vi "FPGAController_v4.vi"() -> ()   [LabVIEW 2015]
uses:
  <vilib>/Utility/miscctls.llb/LVPointTypeDef.ctl
  <vilib>/FPGAPlugInAG/PXIe-7971R/niLvFpga_Open_PXIe-7971R.vi
  <userlib>/_OpenG.lib/comparison/comparison.llb/DBL Changed__ogtk.vi
  <userlib>/_OpenG.lib/file/file.llb/Strip Path Extension - Path__ogtk.vi
  <userlib>/_OpenG.lib/comparison/comparison.llb/Boolean Changed__ogtk.vi
  <vilib>/Utility/error.llb/Error Cluster From Error Code.vi
  <vilib>/rvi/errors/niLvFpgaAdjustHostInterfaceError.vi
  <vilib>/addons/database/Connection.llb/Conn Execute.vi
  <vilib>/addons/database/Recordset.llb/Rec Fetch Recordset Data (R).vi
  <vilib>/addons/database/Recordset.llb/Rec Destroy - Connection.vi
  <vilib>/FPGAPlugInAG/PXIe-7971R/niLvFpga_Close_PXIe-7971R.vi
  <vilib>/rvi/interface/nirviOpenFPGA/nirviOpenFPGA.xnode
  FPGA Bitfiles/FPGA2_FPGATarget_FPGAcode_ccKM5CyXNW8.lvbitx
  <vilib>/rvi/interface/nirviMethod/nirviMethod.xnode
  <vilib>/FPGA/interface/niFpgaViExecutionMode.ctl
  <vilib>/rvi/interface/nirviReadWriteControl/nirviReadWriteControl.xnode
  <vilib>/addons/database/_DB Variant To Data/Database Variant To Data.xnode
  <vilib>/rvi/interface/nirviCloseFPGA/nirviCloseFPGA.xnode
  <vilib>/addons/database/NI_Database_API.lvlib
  NiFpgaLv.dll
panel:
  out "Time Betwee Shots":dbl
  out "Del Armed":bool
  in  "Lower Threshold":bool
  in  "Raise Threshold":bool
  out "Update Threshold":bool
  in  "Min. Time\nBetween Shots (s)":dbl
  in  "Rate Limiting":bool
  out "Armed":bool
  in  "Add Delay":bool
  in  "Delay Name":string
  in  "Delay Value":dbl=3.0 min=0.0
  in  "Delay Ring":dbl(ring)=3.15039 items=["Ablation Chamber"=6.45, "LEIL Chamber"=4.318, "Third Detector"=3.15039, "Custom"=0.0]
  in  "Rearm Trigger":bool
  in  "One Shot Mode":bool
  out "Last Update:":timestamp
  out "Updating FPGA":bool
  out "Sensitivity":dbl
  out "error out":errorcluster
  out "Low Mass Limit":fxp<+,31,17>
  out "High Mass Limit":fxp<+,31,17>
  out "stopping":bool
  in  "Auto Threshold":bool
  out "Peletron (MV)":dbl=2.0
  out "High Mass (kg)":dbl=inf
  out "Low Mass (kg)":dbl
  out "High Charge Limit":i16
  out "Low Charge Limit":i16
  out "High velocity count":i32=210
  out "Low velocity count":i32=21000
  in  "stop":bool
  in  "Peak-Threshold Factor":dbl=2.0
  out "Low Charge Limit (fC)":dbl
  out "High Charge Limit (fC)":dbl=100.0
  out "High Velocity":dbl=100000.0
  out "Low Velocity":dbl=1000.0
  out "Filter 7 Peak":i32=7483
  out "Filter 6 Peak":i32=9863
  out "Filter 5 Peak":i32=13910
  out "Filter 4 Peak":i32=18191
  out "Filter 3 Peak":i32=46254
  out "Filter 2 Peak":i32=120664
  out "Filter 1 Peak":i32=295996
  in  "Filter7 Threshold":i32=-21165
  in  "Filter6 Threshold":i32=-29358
  in  "Filter5 Threshold":i32=-41730
  in  "Filter4 Threshold":i32=-54306
  in  "Filter3 Threshold":i32=-138762
  in  "Filter2 Threshold":i32=-361992
  in  "Filter1 Threshold":i32=-887988
  in  "Zero Peak Values":bool
  in  "Assign Threshold":bool
  in  "Run Mode":bool
  # "Settings"
  # "Dubugging"
  # "Independent Variable"
  # "Low Vel."
  # "High Vel."
  # "Low Q (fC)"
  # "High Q (fC)"
  # "Plate Control While Loop Counter"
  # "Low Mass (kg)"
  # "High Mass (kg)"
  # "Sens. (V/pC)"
  # "Peletron (MV)"
  # "Current Value of Running Average"
  # "Peak Threshold Factor"
  # "Delay Trigger"
  # "Dist. from 2nd Det. (m)"
  # "Name"
  # "Peak Values"
  # "Peak 1"
  # "Peak 2"
  # "Peak 3"
  # "Peak 4"
  # "Peak 5"
  # "Peak 6"
  # "Peak 7"
  # "Thresholds"
  # "Threshold 1"
  # "Threshold 2"
  # "Threshold 3"
  # "Threshold 4"
  # "Threshold 5"
  # "Threshold 6"
  # "Threshold 7"
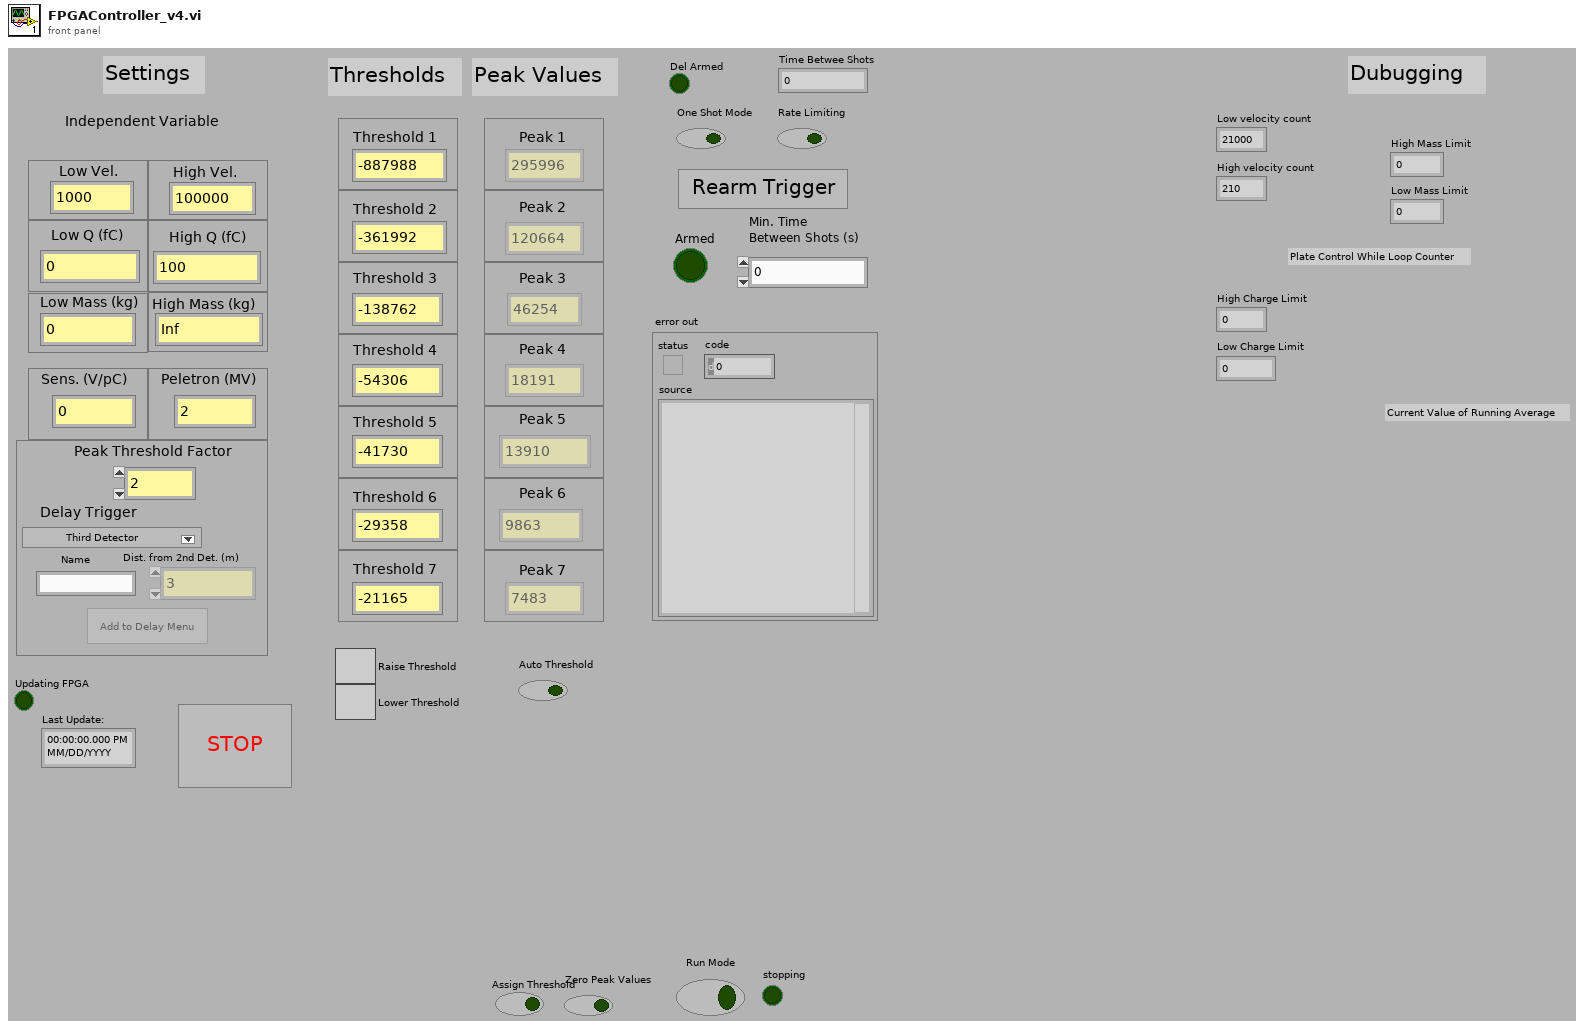
[diagram p1: front panel]
types:
  T1 = typedef "LVPointTypeDef.ctl" = cluster{"Horizontal":i16, "Vertical":i16}
  T2 = enum8{"Enabled", "Disabled", "Disabled and Grayed Out"}
  T3 = typedef "NI_Database_API.lvlib/Conn ObjectReference.ctl" = refnum<k1>
  T4 = cluster{"Filter 1 Peak":i32, "Filter 2 Peak":i32, "Filter 3 Peak":i32, "Filter 4 Peak":i32, "Filter 5 Peak":i32, "Filter 6 Peak":i32, "Filter 7 Peak":i32}
  T5 = typedef "NI_Database_API.lvlib/Rec ObjectReference.ctl" = refnum<k1>
  T6 = typedef "LVStringsAndValuesArrayTypeDef_DBL.ctl" = cluster{"String":string, "Value":dbl}[]
  T7 = cluster{"Numeric":dbl, "Numeric":dbl, "Numeric":dbl, "Numeric":dbl, "Numeric":dbl, "Numeric":dbl, dbl, dbl, "Value":dbl, fxp<+,16,7>, bool}
  T8 = cluster{"Low Velocity Count":i32, "High Velocity Count":i32, "Low Charge Limit (ADC ticks)":i16, "High Charge Limit (ADC ticks)":i16, "Low Mass (ADC*cycle^2)":i64, "High Mass (ADC*cycle^2)":i64, "Mult":fxp<+,16,7>, "Mult Use?":bool}
  T9 = cluster{"Filter 1 Detector 3 Correlation":i32, "Filter 2 Detector 3 Correlation":i32, "Filter 3 Detector 3 Correlation":i32, "Filter 4 Detector 3 Correlation":i32, "Filter 5 Detector 3 Correlation":i32, "Filter 6 Detector 3 Correlation":i32, "Filter 7 Detector 3 Correlation":i32}
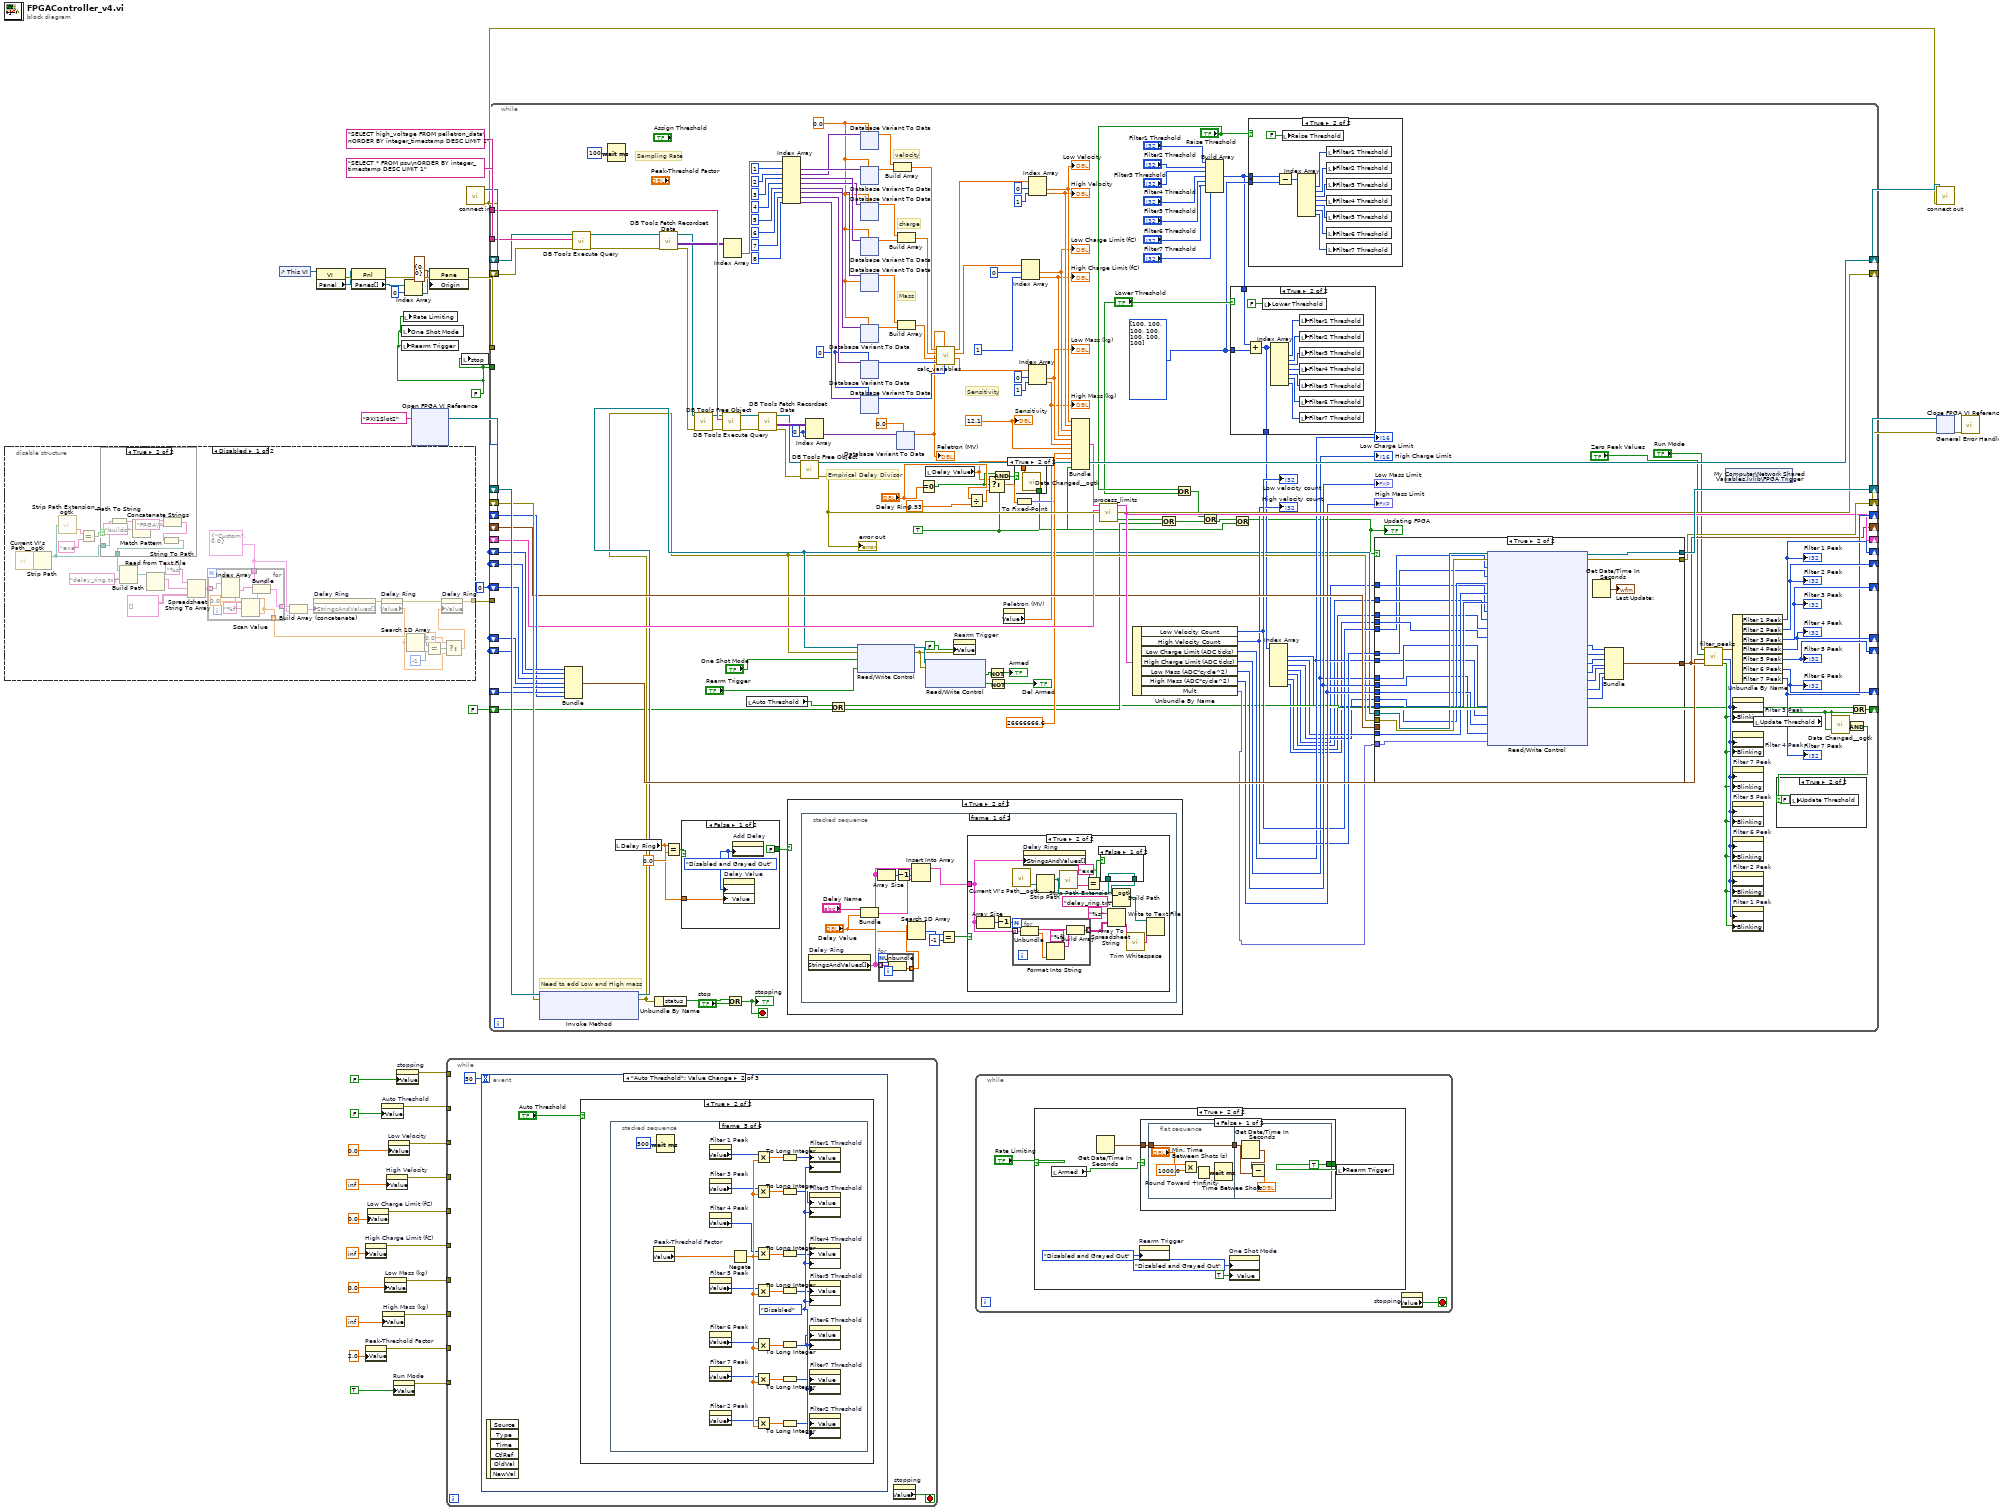
[diagram p0: block diagram]
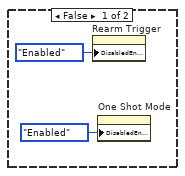
[diagram p4: hidden frame]
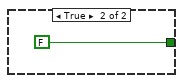
[diagram p5: hidden frame]
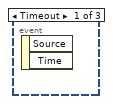
[diagram p6: hidden frame]
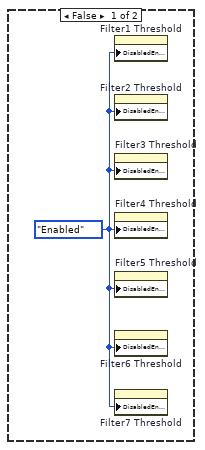
[diagram p7: hidden frame]
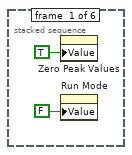
[diagram p8: hidden frame]
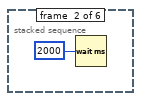
[diagram p9: hidden frame]
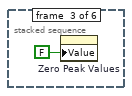
[diagram p10: hidden frame]
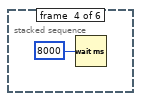
[diagram p11: hidden frame]
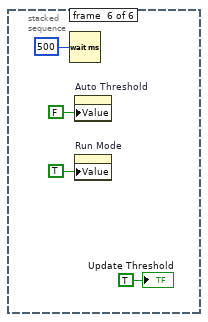
[diagram p12: hidden frame]
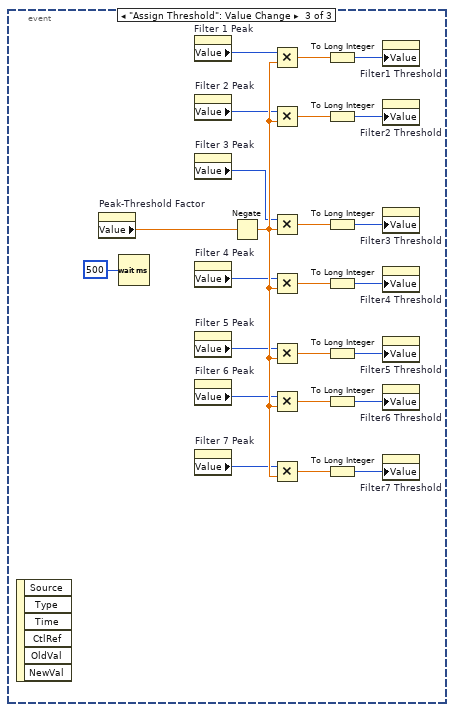
[diagram p13: hidden frame]
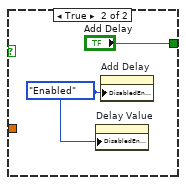
[diagram p18: hidden frame]
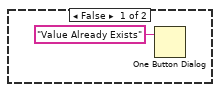
[diagram p20: hidden frame]
diagram:
  w1 = FALSE
  w42 = 0
  n1 = disable-structure shown="Disabled" {
    disable-tunnel: [w50 _] -> w3
    frame Disabled {
      w59 = cluster{"String":string, "Value":dbl} {"String"="Custom", "Value"=0.0}
      n2 = call <userlib>:"Current VI's Path__ogtk.vi"() -> ("Current VI's Path (+ Relative)"=w68:path)  [unwired: 1 in]
      n3 = Strip Path(path=w68) -> (stripped path=w54:path)  [unwired: 1 out]
      n4 = call-poly <userlib>:"Strip Path Extension__ogtk.vi"("path"=w54) -> ("extension"=w58:string)  [unwired: 1 out]
      n5 = Equal?(x=w58, y="exe") -> (x = y?=w55:bool)
      n6 = case shown="True" w55 {
        tunnel: w54 -> [w77 w84]
        tunnel: [w77 w78] -> w53
        frame False {
        }
        frame True {
          n7 = Path To String(path=w84) -> (string=w83:string)
          n8 = Match Pattern(string=w83, regular expression="builds") -> (before substring=w81:string)  [unwired: 1 in, 3 out]
          n9 = Concatenate Strings(w81, "FPGA\\" ("string")) -> (w79:string)
          n10 = String To Path(string=w79) -> (path=w78:path)
        }
      }
      n11 = Build Path(base path=w53, name or relative path="delay_ring.txt") -> (appended path=w56:path)
      n12 = Read from Text File(file (use dialog)=w56) -> (text=w66:string)  [unwired: 3 in, 3 out]
      n13 = Spreadsheet String To Array(format string="%s", spreadsheet string=w66, array type (2D Dbl)=string[][] []) -> (array=w63:string[][])  [unwired: 1 in]
      n14 = for {
        tunnel: w63 -> [w76] mode=indexing
        tunnel: w59 -> [w74]
        tunnel: [w70] -> w60 mode=indexing
        tunnel: [w69] -> w52 mode=indexing
        n15 = Index Array(array=w76) -> (element #1=w75:string, element #2=w73:string)  [unwired: 2 in]
        n16 = Scan Value(string=w73, format string="%f", default (0 dbl)=0.0) -> (value=w69:dbl)  [unwired: 1 out]
        n17 = Bundle(cluster=w74, "String"=w75, "Value"=w69) -> (w70:cluster{"String":string, "Value":dbl})
      }
      n18 = Build Array (concatenate)(w60, w59) -> (w62:cluster{"String":string, "Value":dbl}[])
      n19 = property on="Delay Ring" class="Ring (strict)"("StringsAndValues[]"=w62) -> (error out=w61:errorcluster)  [unwired: 2 in, 1 out]
      n20 = property on="Delay Ring" class="Ring (strict)"(error in=w61) -> (error out=w51:errorcluster, "Value"=w45:dbl)  [unwired: 1 in, 1 out]
      n21 = Search 1D Array(1D array=w52, element=w45) -> (index of element=w49:i32)  [unwired: 1 in]
      n22 = Equal?(x=w49, y=-1) -> (x = y?=w47:bool)
      n23 = Select(t=0.0, s=w47, f=w45) -> (s? t:f=w46:dbl)
      n24 = property on="Delay Ring" class="Ring (strict)"(error in=w51, "Value"=w46) -> (error out=w50:errorcluster)  [unwired: 1 in, 1 out]
    }
    frame Enabled {
    }
  }
  n25 = control-ref of="This VI"() -> (w14:refnum<vi>)
  n26 = property class="VI"(reference=w14) -> (error out=w13:errorcluster, "Panel"=w12:refnum<vi>)  [unwired: 1 in, 1 out]
  n27 = property class="Pnl"(reference=w12, error in=w13) -> (error out=w11:errorcluster, "Panes[]"=w10:refnum<vi>[])  [unwired: 1 out]
  n28 = property on="High Charge Limit (fC)" class="DigNum (strict)"("Value"=inf ("High Charge Limit (fC)")) -> (error out=w29:errorcluster)  [unwired: 2 in, 1 out]
  n29 = property on="Peak-Threshold Factor" class="DigNum (strict)"("Value"=2.0 ("Peak-Threshold Factor")) -> (error out=w23:errorcluster)  [unwired: 2 in, 1 out]
  n30 = property on="Low Charge Limit (fC)" class="DigNum (strict)"("Value"=0.0 ("Low Charge Limit (fC)")) -> (error out=w31:errorcluster)  [unwired: 2 in, 1 out]
  n31 = property on="Auto Threshold" class="Bool (strict)"("Value"=FALSE ("Auto Threshold")) -> (error out=w37:errorcluster)  [unwired: 2 in, 1 out]
  n32 = property on="High Mass (kg)" class="DigNum (strict)"("Value"=inf ("High Mass (kg)")) -> (error out=w25:errorcluster)  [unwired: 2 in, 1 out]
  n33 = property on="Low Mass (kg)" class="DigNum (strict)"("Value"=0.0 ("Low Mass (kg)")) -> (error out=w27:errorcluster)  [unwired: 2 in, 1 out]
  n34 = property on="High Velocity" class="DigNum (strict)"("Value"=inf ("High Velocity")) -> (error out=w33:errorcluster)  [unwired: 2 in, 1 out]
  n35 = property on="Low Velocity" class="DigNum (strict)"("Value"=0.0 ("Low Velocity")) -> (error out=w35:errorcluster)  [unwired: 2 in, 1 out]
  n36 = property on="Run Mode" class="Bool (strict)"("Value"=TRUE ("Run Mode")) -> (error out=w21:errorcluster)  [unwired: 2 in, 1 out]
  n37 = property on="stopping" class="Bool (strict)"("Value"=FALSE ("stopping")) -> (error out=w39:errorcluster)  [unwired: 2 in, 1 out]
  n38 = local write "Rearm Trigger"(w1) -> ()
  n39 = local write "One Shot Mode"(w1) -> ()
  n40 = local write "Rate Limiting"(w1) -> ()
  n41 = Index Array(array=w10, index=0) -> (element=w8:refnum<vi>)
  n42 = xnode "Open FPGA VI Reference"("resource name"=tag "PXI1Slot2") -> ("FPGA VI Reference Out"=w5:refnum<k20>)  [unwired: 1 in, 1 out]
  n43 = property class="Pane"(reference=w8, error in=w11, "Origin"=T1 {"Horizontal"=0, "Vertical"=0}) -> (error out=w6:errorcluster)  [unwired: 1 out]
  n44 = while {
    tunnel: w39 -> [_]
    tunnel: w37 -> [_]
    tunnel: w35 -> [_]
    tunnel: w33 -> [_]
    tunnel: w31 -> [_]
    tunnel: w29 -> [_]
    tunnel: w27 -> [_]
    tunnel: w25 -> [_]
    tunnel: w23 -> [_]
    tunnel: w21 -> [_]
    stop <- w86 stop-if-true
    n45 = event shown="[1] \"Auto Threshold\": Value Change" {
      selector: _ -> [_ _ _]
      dyn-events: _ -> [_ _ _]
      timeout: 50 -> [_ _ _]
      event Timeout {
        n46 = event-data() -> ()  [unwired: 1 in, 2 out]
      }
      event "Auto Threshold": Value Change {
        n47 = event-data() -> ()  [unwired: 1 in, 6 out]
        n48 = case shown="True" "Auto Threshold" {
          frame False {
            w88 = T2."Enabled" ("Disabled")
            n49 = property on="Filter1 Threshold" class="DigNum (strict)"("DisabledEnum"=w88) -> ()  [unwired: 2 in, 2 out]
            n50 = property on="Filter2 Threshold" class="DigNum (strict)"("DisabledEnum"=w88) -> ()  [unwired: 2 in, 2 out]
            n51 = property on="Filter3 Threshold" class="DigNum (strict)"("DisabledEnum"=w88) -> ()  [unwired: 2 in, 2 out]
            n52 = property on="Filter4 Threshold" class="DigNum (strict)"("DisabledEnum"=w88) -> ()  [unwired: 2 in, 2 out]
            n53 = property on="Filter5 Threshold" class="DigNum (strict)"("DisabledEnum"=w88) -> ()  [unwired: 2 in, 2 out]
            n54 = property on="Filter6 Threshold" class="DigNum (strict)"("DisabledEnum"=w88) -> ()  [unwired: 2 in, 2 out]
            n55 = property on="Filter7 Threshold" class="DigNum (strict)"("DisabledEnum"=w88) -> ()  [unwired: 2 in, 2 out]
          }
          frame True {
            n56 = stacked-sequence {
              frame #0 {
                n57 = property on="Zero Peak Values" class="Bool (strict)"("Value"=TRUE ("Zero Peak Values")) -> ()  [unwired: 2 in, 2 out]
                n58 = property on="Run Mode" class="Bool (strict)"("Value"=FALSE ("Run Mode")) -> ()  [unwired: 2 in, 2 out]
              }
              frame #1 {
                n59 = Wait (ms)(milliseconds to wait=u32 2000) -> ()  [unwired: 1 out]
              }
              frame #2 {
                n60 = property on="Zero Peak Values" class="Bool (strict)"("Value"=FALSE ("Zero Peak Values")) -> ()  [unwired: 2 in, 2 out]
              }
              frame #3 {
                n61 = Wait (ms)(milliseconds to wait=u32 8000) -> ()  [unwired: 1 out]
              }
              frame #4 {
                w118 = T2."Disabled" ("Disabled")
                n62 = property on="Peak-Threshold Factor" class="DigNum (strict)"() -> ("Value"=w103:dbl)  [unwired: 2 in, 2 out]
                n63 = Wait (ms)(milliseconds to wait=u32 500) -> ()  [unwired: 1 out]
                n64 = property on="Filter 1 Peak" class="DigNum (strict)"() -> ("Value"=w101:i32)  [unwired: 2 in, 2 out]
                n65 = property on="Filter 3 Peak" class="DigNum (strict)"() -> ("Value"=w99:i32)  [unwired: 2 in, 2 out]
                n66 = property on="Filter 4 Peak" class="DigNum (strict)"() -> ("Value"=w98:i32)  [unwired: 2 in, 2 out]
                n67 = property on="Filter 5 Peak" class="DigNum (strict)"() -> ("Value"=w97:i32)  [unwired: 2 in, 2 out]
                n68 = property on="Filter 6 Peak" class="DigNum (strict)"() -> ("Value"=w96:i32)  [unwired: 2 in, 2 out]
                n69 = property on="Filter 7 Peak" class="DigNum (strict)"() -> ("Value"=w95:i32)  [unwired: 2 in, 2 out]
                n70 = property on="Filter 2 Peak" class="DigNum (strict)"() -> ("Value"=w100:i32)  [unwired: 2 in, 2 out]
                n71 = Negate(x=w103) -> (-x=w102:dbl)
                n72 = Multiply(x=w101, y=w102) -> (x*y=w117:dbl)
                n73 = Multiply(x=w99, y=w102) -> (x*y=w113:dbl)
                n74 = Multiply(x=w98, y=w102) -> (x*y=w111:dbl)
                n75 = Multiply(x=w97, y=w102) -> (x*y=w109:dbl)
                n76 = Multiply(x=w96, y=w102) -> (x*y=w107:dbl)
                n77 = Multiply(x=w95, y=w102) -> (x*y=w105:dbl)
                n78 = Multiply(x=w100, y=w102) -> (x*y=w115:dbl)
                n79 = To Long Integer(number=w117) -> (32bit integer=w116:i32)
                n80 = To Long Integer(number=w113) -> (32bit integer=w112:i32)
                n81 = To Long Integer(number=w111) -> (32bit integer=w110:i32)
                n82 = To Long Integer(number=w109) -> (32bit integer=w108:i32)
                n83 = To Long Integer(number=w107) -> (32bit integer=w106:i32)
                n84 = To Long Integer(number=w105) -> (32bit integer=w104:i32)
                n85 = To Long Integer(number=w115) -> (32bit integer=w114:i32)
                n86 = property on="Filter1 Threshold" class="DigNum (strict)"("Value"=w116, "DisabledEnum"=w118) -> ()  [unwired: 2 in, 2 out]
                n87 = property on="Filter3 Threshold" class="DigNum (strict)"("Value"=w112, "DisabledEnum"=w118) -> ()  [unwired: 2 in, 2 out]
                n88 = property on="Filter4 Threshold" class="DigNum (strict)"("Value"=w110, "DisabledEnum"=w118) -> ()  [unwired: 2 in, 2 out]
                n89 = property on="Filter5 Threshold" class="DigNum (strict)"("Value"=w108, "DisabledEnum"=w118) -> ()  [unwired: 2 in, 2 out]
                n90 = property on="Filter6 Threshold" class="DigNum (strict)"("Value"=w106, "DisabledEnum"=w118) -> ()  [unwired: 2 in, 2 out]
                n91 = property on="Filter7 Threshold" class="DigNum (strict)"("Value"=w104, "DisabledEnum"=w118) -> ()  [unwired: 2 in, 2 out]
                n92 = property on="Filter2 Threshold" class="DigNum (strict)"("Value"=w114, "DisabledEnum"=w118) -> ()  [unwired: 2 in, 2 out]
              }
              frame #5 {
                n93 = Wait (ms)(milliseconds to wait=u32 500) -> ()  [unwired: 1 out]
                n94 = property on="Auto Threshold" class="Bool (strict)"("Value"=FALSE ("Auto Threshold")) -> ()  [unwired: 2 in, 2 out]
                n95 = property on="Run Mode" class="Bool (strict)"("Value"=TRUE ("Run Mode")) -> ()  [unwired: 2 in, 2 out]
                "Update Threshold" <- TRUE ("Update Threshold")
              }
            }
          }
        }
      }
      event "Assign Threshold": Value Change {
        n96 = event-data() -> ()  [unwired: 1 in, 6 out]
        n97 = property on="Peak-Threshold Factor" class="DigNum (strict)"() -> ("Value"=w137:dbl)  [unwired: 2 in, 2 out]
        n98 = Wait (ms)(milliseconds to wait=u32 500) -> ()  [unwired: 1 out]
        n99 = property on="Filter 1 Peak" class="DigNum (strict)"() -> ("Value"=w136:i32)  [unwired: 2 in, 2 out]
        n100 = property on="Filter 2 Peak" class="DigNum (strict)"() -> ("Value"=w135:i32)  [unwired: 2 in, 2 out]
        n101 = property on="Filter 3 Peak" class="DigNum (strict)"() -> ("Value"=w134:i32)  [unwired: 2 in, 2 out]
        n102 = property on="Filter 4 Peak" class="DigNum (strict)"() -> ("Value"=w133:i32)  [unwired: 2 in, 2 out]
        n103 = property on="Filter 5 Peak" class="DigNum (strict)"() -> ("Value"=w132:i32)  [unwired: 2 in, 2 out]
        n104 = property on="Filter 6 Peak" class="DigNum (strict)"() -> ("Value"=w131:i32)  [unwired: 2 in, 2 out]
        n105 = property on="Filter 7 Peak" class="DigNum (strict)"() -> ("Value"=w130:i32)  [unwired: 2 in, 2 out]
        n106 = Negate(x=w137) -> (-x=w139:dbl)
        n107 = Multiply(x=w136, y=w139) -> (x*y=w146:dbl)
        n108 = Multiply(x=w135, y=w139) -> (x*y=w144:dbl)
        n109 = Multiply(x=w134, y=w139) -> (x*y=w143:dbl)
        n110 = Multiply(x=w133, y=w139) -> (x*y=w142:dbl)
        n111 = Multiply(x=w132, y=w139) -> (x*y=w141:dbl)
        n112 = Multiply(x=w131, y=w139) -> (x*y=w140:dbl)
        n113 = Multiply(x=w130, y=w139) -> (x*y=w145:dbl)
        n114 = To Long Integer(number=w146) -> (32bit integer=w129:i32)
        n115 = To Long Integer(number=w144) -> (32bit integer=w128:i32)
        n116 = To Long Integer(number=w143) -> (32bit integer=w127:i32)
        n117 = To Long Integer(number=w142) -> (32bit integer=w126:i32)
        n118 = To Long Integer(number=w141) -> (32bit integer=w125:i32)
        n119 = To Long Integer(number=w140) -> (32bit integer=w124:i32)
        n120 = To Long Integer(number=w145) -> (32bit integer=w123:i32)
        n121 = property on="Filter1 Threshold" class="DigNum (strict)"("Value"=w129) -> ()  [unwired: 2 in, 2 out]
        n122 = property on="Filter2 Threshold" class="DigNum (strict)"("Value"=w128) -> ()  [unwired: 2 in, 2 out]
        n123 = property on="Filter3 Threshold" class="DigNum (strict)"("Value"=w127) -> ()  [unwired: 2 in, 2 out]
        n124 = property on="Filter4 Threshold" class="DigNum (strict)"("Value"=w126) -> ()  [unwired: 2 in, 2 out]
        n125 = property on="Filter5 Threshold" class="DigNum (strict)"("Value"=w125) -> ()  [unwired: 2 in, 2 out]
        n126 = property on="Filter6 Threshold" class="DigNum (strict)"("Value"=w124) -> ()  [unwired: 2 in, 2 out]
        n127 = property on="Filter7 Threshold" class="DigNum (strict)"("Value"=w123) -> ()  [unwired: 2 in, 2 out]
      }
    }
    n128 = property on="stopping" class="Bool (strict)"() -> ("Value"=w86:bool)  [unwired: 2 in, 2 out]
  }
  n129 = local write "stop"(w1) -> ()
  n130 = call "connect in.vi"() -> ("error out"=w15:errorcluster, "Database Connection"=w16:T3)  [unwired: 7 in, 1 out]
  n131 = while {
    shift-right: [w308] -> w41
    shift-left: w5 -> [w312]
    shift-right: [w307] -> w40
    shift-left: _ -> [w311]
    shift-right: [w303] -> _
    shift-left: w42 -> [w296]
    shift-right: [w302] -> _
    shift-left: w42 -> [w295]
    shift-right: [w301] -> _
    shift-left: w42 -> [w294]
    shift-right: [w300] -> _
    shift-left: w42 -> [w293]
    shift-right: [w299] -> _
    shift-left: w42 -> [w292]
    shift-right: [w305] -> _
    shift-left: w42 -> [w298]
    shift-right: [w304] -> _
    shift-left: w42 -> [w297]
    tunnel: "SELECT * FROM psu\nORDER BY integer_timestamp DESC LIMIT 1" ("SQL query") -> [w291]
    tunnel: "SELECT high_voltage FROM pelletron_data\nORDER BY integer_timestamp DESC LIMIT 1" ("SQL query") -> [w290]
    shift-right: [w286] -> w17
    shift-left: w16 -> [w289]
    shift-right: [w287] -> _
    shift-left: w15 -> [w288]
    shift-right: [w285] -> _
    shift-left: _ -> [w284]
    shift-right: [w282] -> _
    shift-left: _ -> [w283]
    tunnel: w6 -> [_]
    tunnel: w3 -> [_]
    shift-right: [w186] -> _
    shift-left: FALSE -> [w189]
    tunnel: w1 -> [_]
    stop <- w306 stop-if-true
    w148 = i32[] [100, 100, 100, 100, 100, 100, 100]
    w151 = TRUE
    w238 = 0 ("index (row)")
    w246 = i8 0
    w247 = 0.0
    w212 = 12.1
    # "charge"
    # "Empirical Delay Divisor"
    # "Mass"
    # "velocity"
    # "Sensitivity"
    # "Sampling Rate"
    # "Need to add Low and High mass"
    n132 = xnode "Invoke Method"("FPGA VI Reference In"=w312, "error in"=w311) -> ("FPGA VI Reference Out"=w206:refnum<k20>, "error out"=w205:errorcluster)  [unwired: 1 out]
    n133 = Bundle("Filter 1 Peak"=w298, "Filter 2 Peak"=w297, "Filter 3 Peak"=w296, "Filter 4 Peak"=w295, "Filter 5 Peak"=w294, "Filter 6 Peak"=w293, "Filter 7 Peak"=w292) -> (w278:T4)  [unwired: 1 in]
    n134 = call-poly <vilib>:"DB Tools Execute Query.vi"("error in (no error)"=w288, "SQL query"=w291, "connection reference"=w289) -> ("error out"=w266:errorcluster, "recordset reference"=w267:T5)  [unwired: 5 in]
    n135 = Wait (ms)(milliseconds to wait=u32 100) -> ()  [unwired: 1 out]
    n136 = local read "Delay Ring"() -> (w190:dbl)
    n137 = Unbundle By Name(w205) -> ("status"=w310:bool)
    n138 = call-poly <vilib>:"DB Tools Fetch Recordset Data.vi"("error in (no error)"=w266, "recordset reference"=w267) -> ("error out"=w244:errorcluster, "recordset data"=w257:variant[][], "recordset reference out"=w245:T5)  [unwired: 3 in]
    n139 = Equal?(x=w190, y=0.0) -> (x = y?=w191:bool)
    n140 = case shown="False" w191 {
      tunnel: [FALSE ("Add Delay") "Add Delay"] -> w209
      tunnel: w190 -> [w341 _]
      frame False {
        w342 = T2."Disabled and Grayed Out" ("Disabled")
        n141 = property on="Delay Value" class="DigNum (strict)"("DisabledEnum"=w342, "Value"=w341) -> ()  [unwired: 2 in, 2 out]
        n142 = property on="Add Delay" class="Bool (strict)"("DisabledEnum"=w342) -> ()  [unwired: 2 in, 2 out]
      }
      frame True {
        w343 = T2."Enabled" ("Disabled")
        n143 = property on="Delay Value" class="DigNum (strict)"("DisabledEnum"=w343) -> ()  [unwired: 2 in, 2 out]
        n144 = property on="Add Delay" class="Bool (strict)"("DisabledEnum"=w343) -> ()  [unwired: 2 in, 2 out]
      }
    }
    n145 = call-poly <vilib>:"DB Tools Free Object.vi"("error in (no error)"=w244, "recordset reference"=w245) -> ("error out"=w242:errorcluster, "connection reference"=w243:T3)  [unwired: 8 in]
    n146 = call-poly <vilib>:"DB Tools Execute Query.vi"("error in (no error)"=w242, "SQL query"=w290, "connection reference"=w243) -> ("error out"=w240:errorcluster, "recordset reference"=w241:T5)  [unwired: 5 in]
    n147 = Index Array(array=w257) -> (element=w256:variant[])  [unwired: 2 in]
    n148 = Or(x=w310, y="stop") -> (x .or. y?=w306:bool)
    "stopping" <- w306
    n149 = local read "Auto Threshold"() -> (w187:bool)
    n150 = call-poly <vilib>:"DB Tools Fetch Recordset Data.vi"("error in (no error)"=w240, "recordset reference"=w241) -> ("error out"=w213:errorcluster, "recordset data"=w239:variant[][], "recordset reference out"=w214:T5)  [unwired: 3 in]
    n151 = Index Array(array=w256, index #1=1 ("index"), index #2=2 ("index"), index #3=3 ("index"), index #4=4 ("index"), index #5=5 ("index"), index #6=6 ("index"), index #7=7 ("index"), index #8=8 ("index")) -> (element #1=w255:variant, element #2=w254:variant, element #3=w253:variant, element #4=w252:variant, element #5=w251:variant, element #6=w250:variant, element #7=w249:variant, element #8=w248:variant)
    n152 = case shown="True" w209 {
      frame False {
      }
      frame True {
        n153 = stacked-sequence {
          frame #0 {
            n154 = property on="Delay Ring" class="Ring (strict)"() -> ("StringsAndValues[]"=w347:T6)  [unwired: 2 in, 2 out]
            n155 = Bundle("Delay Name"="Delay Name", "Delay Value"="Delay Value") -> (w352:cluster{"Delay Name":string, "Delay Value":dbl})  [unwired: 1 in]
            n156 = Array Size(array=w347) -> (size(s)=w350:i32)
            n157 = for {
              tunnel: w347 -> [w357] mode=indexing
              tunnel: [w356] -> w346 mode=indexing
              n158 = Unbundle(w357) -> ("Value"=w356:dbl)  [unwired: 1 out]
            }
            n159 = Decrement(x=w350) -> (x-1=w349:i32)
            n160 = Search 1D Array(1D array=w346, element="Delay Value") -> (index of element=w354:i32)  [unwired: 1 in]
            n161 = Insert Into Array(array=w347, index=w349, new element=w352) -> (w351:T6)
            n162 = Equal?(x=w354, y=-1) -> (x = y?=w348:bool)
            n163 = case shown="True" w348 {
              tunnel: w351 -> [_ w366]
              frame False {
                n164 = One Button Dialog(message="Value Already Exists") -> ()  [unwired: 1 in, 1 out]
              }
              frame True {
                n165 = Array Size(array=w366) -> (size(s)=w368:i32)
                n166 = Decrement(x=w368) -> (x-1=w367:i32)
                n167 = call <userlib>:"Current VI's Path__ogtk.vi"() -> ("Current VI's Path (+ Relative)"=w372:path)  [unwired: 1 in]
                n168 = for {
                  N: w367 -> [_]
                  tunnel: w366 -> [w382] mode=indexing
                  tunnel: [w377] -> w369 mode=indexing
                  n169 = Unbundle(w382) -> ("String"=w378:string, "Value"=w381:dbl)
                  n170 = Format Into String(format string="%f", w381) -> (resulting string=w379:string)  [unwired: 2 in, 1 out]
                  n171 = Build Array(w378, w379) -> (w377:string[])
                }
                n172 = property on="Delay Ring" class="Ring (strict)"("StringsAndValues[]"=w366) -> ()  [unwired: 2 in, 2 out]
                n173 = Strip Path(path=w372) -> (stripped path=w360:path)  [unwired: 1 out]
                n174 = call-poly <userlib>:"Strip Path Extension__ogtk.vi"("path"=w360) -> ("extension"=w363:string)  [unwired: 1 out]
                n175 = Equal?(x="exe", y=w363) -> (x = y?=w361:bool)
                n176 = case shown="False" w361 {
                  tunnel: w360 -> [w374 w376]
                  tunnel: [w374 w375] -> w359
                  frame False {
                  }
                  frame True {
                    n177 = Strip Path(path=w376) -> (stripped path=w375:path)  [unwired: 1 out]
                  }
                }
                n178 = Array To Spreadsheet String(array=w369, 3:"%s" ("format string")) -> (spreadsheet string=w365:string)  [unwired: 1 in]
                n179 = Build Path(base path=w359, name or relative path="delay_ring.txt") -> (appended path=w370:path)
                n180 = call <vilib>:"Trim Whitespace.vi"("string"=w365) -> ("trimmed string"=w364:string)  [unwired: 1 in]
                n181 = Write to Text File(file (use dialog)=w370, text=w364) -> ()  [unwired: 2 in, 3 out]
              }
            }
          }
          frame #1 {
            n182 = property on="Add Delay" class="Bool (strict)"("Value"=FALSE ("Add Delay")) -> ()  [unwired: 2 in, 2 out]
          }
        }
      }
    }
    n183 = call-poly <vilib>:"DB Tools Free Object.vi"("error in (no error)"=w213, "recordset reference"=w214) -> ("error out"=w287:errorcluster, "connection reference"=w286:T3)  [unwired: 8 in]
    "error out" <- w287
    n184 = Index Array(array=w239, index (row)=w238, index (col)=w238) -> (element=w237:variant)
    n185 = Or(x=w187, y=w189) -> (x .or. y?=w188:bool)
    n186 = xnode "Read/Write Control"("FPGA VI Reference In"=w206, "error in"=w205, "One Shot"="One Shot Mode", "Reset One Shot"="Rearm Trigger") -> ("FPGA VI Reference Out"=w199:refnum<k20>, "error out"=w198:errorcluster)
    n187 = xnode "Database Variant To Data"("database variant"=w254, "type"=w247) -> ("data"=w162:dbl)  [unwired: 1 in, 1 out]
    n188 = xnode "Database Variant To Data"("database variant"=w255, "type"=w247) -> ("data"=w163:dbl)  [unwired: 1 in, 1 out]
    n189 = xnode "Database Variant To Data"("database variant"=w252, "type"=w247) -> ("data"=w161:dbl)  [unwired: 1 in, 1 out]
    n190 = xnode "Database Variant To Data"("database variant"=w253, "type"=w247) -> ("data"=w160:dbl)  [unwired: 1 in, 1 out]
    n191 = xnode "Database Variant To Data"("database variant"=w250, "type"=w247) -> ("data"=w159:dbl)  [unwired: 1 in, 1 out]
    n192 = xnode "Database Variant To Data"("database variant"=w251, "type"=w247) -> ("data"=w158:dbl)  [unwired: 1 in, 1 out]
    n193 = xnode "Database Variant To Data"("database variant"=w249, "type"=w246) -> ("data"=w231:i8)  [unwired: 1 in, 1 out]
    n194 = xnode "Database Variant To Data"("database variant"=w248, "type"=w246) -> ("data"=w230:i8)  [unwired: 1 in, 1 out]
    n195 = Build Array(w162, w163) -> (w234:dbl[])
    n196 = xnode "Database Variant To Data"("database variant"=w237, "type"=0.0) -> ("data"=w157:dbl)  [unwired: 1 in, 1 out]
    "Peletron (MV)" <- w157
    n197 = Build Array(w161, w160) -> (w233:dbl[])
    n198 = Build Array(w159, w158) -> (w232:dbl[])
    n199 = Equal To 0?(x="Delay Ring") -> (x = 0?=w156:bool)
    n200 = xnode "Read/Write Control"("FPGA VI Reference In"=w199, "error in"=w198) -> ("Not Armed?"=w197:bool, "Del Not Armed?"=w150:bool)  [unwired: 2 out]
    n201 = local read "Delay Value"() -> (w155:dbl)
    n202 = call "calc_variables.vi"("var2"=w230, "Peletron"=w157, "var1"=w231, "Mass"=w232, "Charge"=w233, "Velocity"=w234) -> ("Mass out"=w223:dbl[], "Charge out"=w226:dbl[], "Velocity out"=w229:dbl[])  [unwired: 3 in]
    n203 = property on="Rearm Trigger" class="Bool (strict)"(error in=w198, "Value"=FALSE ("Rearm Trigger")) -> ()  [unwired: 1 in, 2 out]
    n204 = Divide(x="Delay Ring", y=0.93) -> (x/y=w195:dbl)
    n205 = Select(t=w155, s=w156, f=w195) -> (s? t:f=w194:dbl)
    n206 = Not(x=w197) -> (.not. x?=→"Armed":bool)
    n207 = Not(x=w150) -> (.not. x?=→"Del Armed":bool)
    n208 = And(x=w156, y=w151) -> (x .and. y?=w152:bool)
    n209 = property on="Peletron (MV)" class="DigNum (strict)"() -> ("Value"=w235:dbl)  [unwired: 2 in, 2 out]
    n210 = case shown="True" w152 {
      selector: w152 -> [w313 _]
      tunnel: w155 -> [_ w315]
      tunnel: [w313 w314] -> w153
      frame False {
      }
      frame True {
        n211 = call-poly <userlib>:"Data Changed__ogtk.vi"("DBL"=w315) -> ("Changed"=w314:bool)
      }
    }
    n212 = To Fixed-Point(number=w194) -> (fixed-point=w208:fxp<+,16,7>)  [unwired: 1 in]
    n213 = Index Array(array=w226, index #1=0 ("index"), index #2=1 ("index")) -> (element #1=w218:dbl, element #2=w217:dbl)
    "High Charge Limit (fC)" <- w217
    "Low Charge Limit (fC)" <- w218
    n214 = Index Array(array=w229, index #1=0 ("index"), index #2=1 ("index")) -> (element #1=w220:dbl, element #2=w219:dbl)
    "High Velocity" <- w219
    "Low Velocity" <- w220
    n215 = Index Array(array=w223, index #1=0 ("index"), index #2=1 ("index")) -> (element #1=w216:dbl, element #2=w215:dbl)
    "Low Mass (kg)" <- w216
    "High Mass (kg)" <- w215
    n216 = Bundle("Numeric"=w220, "Numeric"=w219, "Numeric"=w218, "Numeric"=w217, "Numeric"=w216, "Numeric"=w215, w212, 26666666.6, "Value"=w235, w208, w151) -> (w277:T7)  [unwired: 1 in]
    n217 = call "process_limits.vi"("old output cluster"=w284, "Input cluster"=w277) -> ("Update FPGA"=w211:bool, "output cluster"=w285:T8)  [unwired: 8 in]
    n218 = Unbundle By Name(w285) -> ("Low Velocity Count"=w273:i32, "High Velocity Count"=w272:i32, "Low Charge Limit (ADC ticks)"=w270:i16, "High Charge Limit (ADC ticks)"=w271:i16, "Low Mass (ADC*cycle^2)"=w275:i64, "High Mass (ADC*cycle^2)"=w276:i64, "Mult"=w207:fxp<+,16,7>)
    "Low velocity count" <- w273
    "High velocity count" <- w272
    "High Charge Limit" <- w271
    "Low Charge Limit" <- w270
    "High Mass Limit" <- w276
    "Low Mass Limit" <- w275
    n219 = Or(x=w211, y=w188) -> (x .or. y?=w193:bool)
    n220 = Or(x="Raise Threshold", y="Lower Threshold") -> (x .or. y?=w164:bool)
    n221 = Or(x=w164, y=w193) -> (x .or. y?=w165:bool)
    n222 = Build Array("Filter1 Threshold", "Filter2 Threshold", "Filter3 Threshold", "Filter4 Threshold", "Filter5 Threshold", "Filter6 Threshold", "Filter7 Threshold") -> (w147:i32[])
    n223 = case shown="True" "Lower Threshold" {
      tunnel: w147 -> [w316 w327]
      tunnel: w148 -> [_ w326]
      tunnel: [w316 w317] -> w178
      frame False {
      }
      frame True {
        n224 = Add(x=w327, y=w326) -> (x+y=w317:i32[])
        n225 = local write "Lower Threshold"(FALSE ("Lower Threshold")) -> ()
        n226 = Index Array(array=w317) -> (element #1=w324:i32, element #2=w323:i32, element #3=w322:i32, element #4=w321:i32, element #5=w320:i32, element #6=w319:i32, element #7=w318:i32)  [unwired: 7 in]
        n227 = local write "Filter1 Threshold"(w324) -> ()
        n228 = local write "Filter2 Threshold"(w323) -> ()
        n229 = local write "Filter3 Threshold"(w322) -> ()
        n230 = local write "Filter4 Threshold"(w321) -> ()
        n231 = local write "Filter5 Threshold"(w320) -> ()
        n232 = local write "Filter6 Threshold"(w319) -> ()
        n233 = local write "Filter7 Threshold"(w318) -> ()
      }
    }
    n234 = Or(x=w165, y=w153) -> (x .or. y?=w154:bool)
    "Updating FPGA" <- w154
    n235 = case shown="True" "Raise Threshold" {
      tunnel: w147 -> [_ w338]
      tunnel: w148 -> [_ w328]
      frame False {
      }
      frame True {
        n236 = Subtract(x=w338, y=w328) -> (x-y=w329:i32[])
        n237 = local write "Raise Threshold"(FALSE ("Raise Threshold")) -> ()
        n238 = Index Array(array=w329) -> (element #1=w336:i32, element #2=w335:i32, element #3=w334:i32, element #4=w333:i32, element #5=w332:i32, element #6=w331:i32, element #7=w330:i32)  [unwired: 7 in]
        n239 = local write "Filter1 Threshold"(w336) -> ()
        n240 = local write "Filter2 Threshold"(w335) -> ()
        n241 = local write "Filter3 Threshold"(w334) -> ()
        n242 = local write "Filter4 Threshold"(w333) -> ()
        n243 = local write "Filter5 Threshold"(w332) -> ()
        n244 = local write "Filter6 Threshold"(w331) -> ()
        n245 = local write "Filter7 Threshold"(w330) -> ()
      }
    }
    n246 = Index Array(array=w178) -> (element #1=w181:i32, element #2=w179:i32, element #3=w176:i32, element #4=w174:i32, element #5=w172:i32, element #6=w170:i32, element #7=w168:i32)  [unwired: 7 in]
    n247 = case shown="True" w154 {
      tunnel: w206 -> [w385 w413]
      tunnel: w205 -> [w386 w412]
      tunnel: [w385 w411] -> w308
      tunnel: [w386 w410] -> w307
      tunnel: w181 -> [_ w409]
      tunnel: w179 -> [_ w408]
      tunnel: w176 -> [_ w407]
      tunnel: w174 -> [_ w406]
      tunnel: w172 -> [_ w405]
      tunnel: w170 -> [_ w404]
      tunnel: w168 -> [_ w403]
      tunnel: [w384 w389] -> w282
      tunnel: w276 -> [_ w395]
      tunnel: w275 -> [_ w394]
      tunnel: w273 -> [_ w393]
      tunnel: w272 -> [_ w392]
      tunnel: w271 -> [_ w391]
      tunnel: w270 -> [_ w390]
      tunnel: w283 -> [w384 _]
      tunnel: w207 -> [_ w387]
      frame False {
      }
      frame True {
        n248 = xnode "Read/Write Control"("FPGA VI Reference In"=w413, "error in"=w412, "Low Velocity Count"=w393, "High Velocity Count"=w392, "Filter 1 threshold"=w409, "Filter 2 threshold"=w408, "Filter 3 threshold"=w407, "Filter 4 threshold"=w406, "Filter 5 threshold"=w405, "Filter 6 threshold"=w404, "Filter 7 threshold"=w403, "High Charge Limit"=w391, "Low Charge Limit"=w390, "High Mass Limit"=w395, "Low Mass Limit"=w394, "Mult1"=w387) -> ("FPGA VI Reference Out"=w411:refnum<k20>, "error out"=w410:errorcluster, "Filter 1 Detector 3 Correlation"=w402:i32, "Filter 2 Detector 3 Correlation"=w401:i32, "Filter 3 Detector 3 Correlation"=w400:i32, "Filter 4 Detector 3 Correlation"=w399:i32, "Filter 5 Detector 3 Correlation"=w398:i32, "Filter 6 Detector 3 Correlation"=w397:i32, "Filter 7 Detector 3 Correlation"=w396:i32)
        n249 = Get Date/Time In Seconds() -> (seconds since 1Jan1904=→"Last Update:":timestamp)
        n250 = Bundle("Filter 1 Detector 3 Correlation"=w402, "Filter 2 Detector 3 Correlation"=w401, "Filter 3 Detector 3 Correlation"=w400, "Filter 4 Detector 3 Correlation"=w399, "Filter 5 Detector 3 Correlation"=w398, "Filter 6 Detector 3 Correlation"=w397, "Filter 7 Detector 3 Correlation"=w396) -> (w389:T9)  [unwired: 1 in]
      }
    }
    n251 = call "filter_peaks.vi"("Correlation cluster"=w282, "Filter peak cluster"=w278, "Zero out"="Zero Peak Values", "Run Mode"="Run Mode") -> ("Blinking"=w269:bool, "status"=w274:T2, "Filter peak output"=w279:T4)  [unwired: 5 in]
    n252 = shared-variable "My Computer\\Network Shared Variables.lvlib\\FPGA Trigger"() -> ()  [unwired: 1 in, 2 out]
    n253 = Unbundle By Name(w279) -> ("Filter 1 Peak"=w305:i32, "Filter 2 Peak"=w304:i32, "Filter 3 Peak"=w303:i32, "Filter 4 Peak"=w302:i32, "Filter 5 Peak"=w301:i32, "Filter 6 Peak"=w300:i32, "Filter 7 Peak"=w299:i32)
    "Filter 1 Peak" <- w305
    "Filter 2 Peak" <- w304
    "Filter 3 Peak" <- w303
    "Filter 4 Peak" <- w302
    "Filter 5 Peak" <- w301
    "Filter 6 Peak" <- w300
    "Filter 7 Peak" <- w299
    n254 = property on="Filter 3 Peak" class="DigNum (strict)"("DisabledEnum"=w274, "Blinking"=w269) -> ()  [unwired: 2 in, 2 out]
    n255 = property on="Filter 4 Peak" class="DigNum (strict)"("DisabledEnum"=w274, "Blinking"=w269) -> ()  [unwired: 2 in, 2 out]
    n256 = property on="Filter 7 Peak" class="DigNum (strict)"("DisabledEnum"=w274, "Blinking"=w269) -> ()  [unwired: 2 in, 2 out]
    n257 = property on="Filter 5 Peak" class="DigNum (strict)"("DisabledEnum"=w274, "Blinking"=w269) -> ()  [unwired: 2 in, 2 out]
    n258 = property on="Filter 6 Peak" class="DigNum (strict)"("DisabledEnum"=w274, "Blinking"=w269) -> ()  [unwired: 2 in, 2 out]
    n259 = property on="Filter 2 Peak" class="DigNum (strict)"("DisabledEnum"=w274, "Blinking"=w269) -> ()  [unwired: 2 in, 2 out]
    n260 = property on="Filter 1 Peak" class="DigNum (strict)"("DisabledEnum"=w274, "Blinking"=w269) -> ()  [unwired: 2 in, 2 out]
    n261 = local read "Update Threshold"() -> (w184:bool)
    n262 = call-poly <userlib>:"Data Changed__ogtk.vi"("Boolean"=w184) -> ("Changed"=w185:bool)
    n263 = And(x=w185, y=w184) -> (x .and. y?=w183:bool)
    n264 = case shown="True" w183 {
      frame False {
      }
      frame True {
        n265 = local write "Update Threshold"(FALSE ("Update Threshold")) -> ()
      }
    }
    n266 = Or(x=w187, y=w184) -> (x .or. y?=w186:bool)
    "Sensitivity" <- w212
  }
  n267 = while {
    stop <- w703 stop-if-true
    n268 = case shown="True" "Rate Limiting" {
      frame False {
        n269 = property on="Rearm Trigger" class="Bool (strict)"("DisabledEnum"=T2."Enabled" ("Disabled")) -> ()  [unwired: 2 in, 2 out]
        n270 = property on="One Shot Mode" class="Bool (strict)"("DisabledEnum"=T2."Enabled" ("Disabled")) -> ()  [unwired: 2 in, 2 out]
      }
      frame True {
        n271 = local read "Armed"() -> (w707:bool)
        n272 = Get Date/Time In Seconds() -> (seconds since 1Jan1904=w706:timestamp)
        n273 = property on="Rearm Trigger" class="Bool (strict)"("DisabledEnum"=T2."Disabled and Grayed Out" ("Disabled")) -> ()  [unwired: 2 in, 2 out]
        n274 = case shown="False" w707 {
          tunnel: [w714 FALSE] -> w711
          tunnel: w706 -> [w713 _]
          frame False {
            n275 = flat-sequence {
              tunnel: w713 -> [w715]
              tunnel: [w715] -> w712
              tunnel: [TRUE] -> w714
              tunnel: w712 -> [w721]
              frame #0 {
                n276 = Multiply(x="Min. Time\nBetween Shots (s)", y=1000.0) -> (x*y=w718:dbl)
                n277 = Round Toward +Infinity(x=w718) -> (ceil(x): smallest int >= x=w716:dbl)
                n278 = Wait (ms)(milliseconds to wait=w716) -> ()  [unwired: 1 out]
              }
              frame #1 {
                n279 = Get Date/Time In Seconds() -> (seconds since 1Jan1904=w722:timestamp)
                n280 = Subtract(x=w722, y=w721) -> (x-y=→"Time Betwee Shots":dbl)
              }
            }
          }
          frame True {
          }
        }
        n281 = property on="One Shot Mode" class="Bool (strict)"("DisabledEnum"=T2."Disabled and Grayed Out" ("Disabled"), "Value"=TRUE ("One Shot Mode")) -> ()  [unwired: 2 in, 2 out]
        n282 = local write "Rearm Trigger"(w711) -> ()
      }
    }
    n283 = property on="stopping" class="Bool (strict)"() -> ("Value"=w703:bool)  [unwired: 2 in, 2 out]
  }
  n284 = call "connect out.vi"("error in (no error)"=w15, "connection reference"=w17) -> ()  [unwired: 9 in, 1 out]
  n285 = xnode "Close FPGA VI Reference"("FPGA VI Reference In"=w41, "error in"=w40) -> ("error out"=w43:errorcluster)
  n286 = call <vilib>:"General Error Handler.vi"("error in (no error)"=w43) -> ()  [unwired: 10 in, 5 out]
